vi "histCase.vi"(0 "CaseControl":T2, 1 "last case":T1, 3 "event":T1, 6 "finish?":bool) -> (14 "CaseControl":T2, 17 "event":T1)   [LabVIEW 2018]
uses:
  TEST/Typedefs/Command.ctl
  Typedefs/CaseControl.ctl
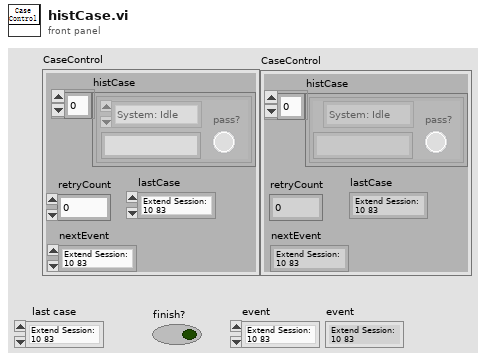
[diagram p1: front panel]
types:
  T1 = typedef "Command.ctl" = enum16{"Extend Session: 10 83", "Tester Present: 3E 80", "Resquest Seed: 27 01", "Send Key: 27 02", "Check FBL:  31 01 FD 02", "Control DTC: 85 82", "Comm Control: 28 83 01", "Program Session Request: 10 02", "Request Seed: 27 35", "Seed Key: 27 36", "Request Download: 34 00 44", "Transfer Data: 36 XX YY", "More Data?", "Request Transfer Exit: 37", "Check Flash Driver Validity: 01 FD 03", "More Segment?", "Write Data Fingereint: 23 F1 F0+26", "EraseFlashMemory Routine: 31 01 FD 00 44", "More segment?(each file)", "CheckAppSwAppData Validity: 31 01 FD 04 44", "CheckAppSwAppData Dependency: 31 01 fd 01", "ECU Reset: 11 81", "System: Init", "System: Idle", "System: Error", "System: Wait", "System: Delay", "System: CAN Send", "System: Exit"}
  T2 = typedef "CaseControl.ctl" = cluster{"histCase":cluster{"time":string, "event":T1, "pass?":bool}[], "retryCount":i32, "lastCase":T1, "nextEvent":T1}
  T3 = cluster{"time":string, "event":T1, "pass?":bool}[]
  T4 = cluster{"time_YMD":string, "  last case":T1, "finish?":bool}
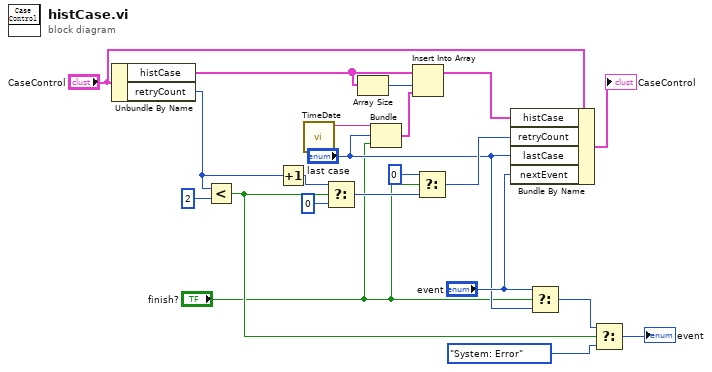
[diagram p0: block diagram]
diagram:
  n1 = Unbundle By Name("CaseControl") -> ("histCase"=w20:T3, "retryCount"=w16:i32)
  n2 = Less?(x=w16, y=2) -> (x < y?=w14:bool)
  n3 = Increment(x=w16) -> (x+1=w12:i32)
  n4 = call "TimeDate.vi"() -> ("time_YMD"=w3:string)  [unwired: 10 in, 1 out]
  n5 = Select(t=w12, s=w14, f=0 ("t")) -> (s? t:f=w7:i32)
  n6 = Array Size(array=w20) -> (size(s)=w21:i32)
  n7 = Bundle("time_YMD"=w3, "last case"="last case", "finish?"="finish?") -> (w4:T4)  [unwired: 1 in]
  n8 = Insert Into Array(array=w20, index=w21, new element=w4) -> (w18:T3)
  n9 = Select(t=0, s="finish?", f=w7) -> (s? t:f=w5:i32)
  n10 = Bundle By Name(cluster="CaseControl", "histCase"=w18, "retryCount"=w5, "lastCase"="last case", "nextEvent"="event") -> (→"CaseControl":T2)
  n11 = Select(t="event", s="finish?", f="last case") -> (s? t:f=w11:T1)
  n12 = Select(t=w11, s=w14, f=Command."System: Error") -> (s? t:f=→"event":T1)
